vi "Get Amp Max Speed.vi"(10 "speed":sgl, 11 "index":i32) -> (2 "speed out":sgl, 3 "function return":u32)   [LabVIEW 2018, in "AndorSDK.lvlib"]
doc: "EXPNETTYPE unsigned int WINAPI GetAmpMaxSpeed(int index, float * speed);"
uses:
  AndorSDK.lvlib
  ATMCD32D.dll
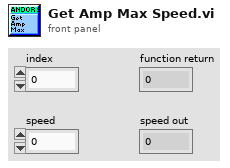
[diagram p1: front panel]
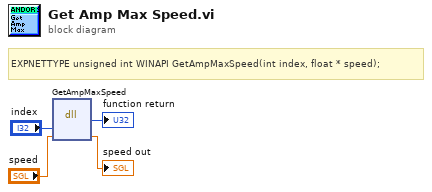
[diagram p0: block diagram]
diagram:
  # "EXPNETTYPE unsigned int WINAPI GetAmpMaxSpeed(int index, float * speed);"
  n1 = dll-call lib="PTH2babs E\nPersönliches02 - Arbeit03-HiwijobsLabviewCodelibANDOR\tAndor SDK\nATMCD32D.*" fn="GetAmpMaxSpeed"("index"="index", "speed"="speed") -> (→"function return":u32, "speed"=→"speed out":sgl)  [unwired: 4 in, 2 out]
